vi "LoadPosMove.vi"(11 "UiDefinition":T1) -> ()   [LabVIEW 2020]
uses:
  UIReferences.ctl
  C:/Users/User/Desktop/Automation/CurrentVersion/LabviewDXFViewer/bin/Release/LabviewDXFViewer.exe
  LabviewDXFViewer/bin/Release/LabviewDXFViewer.exe
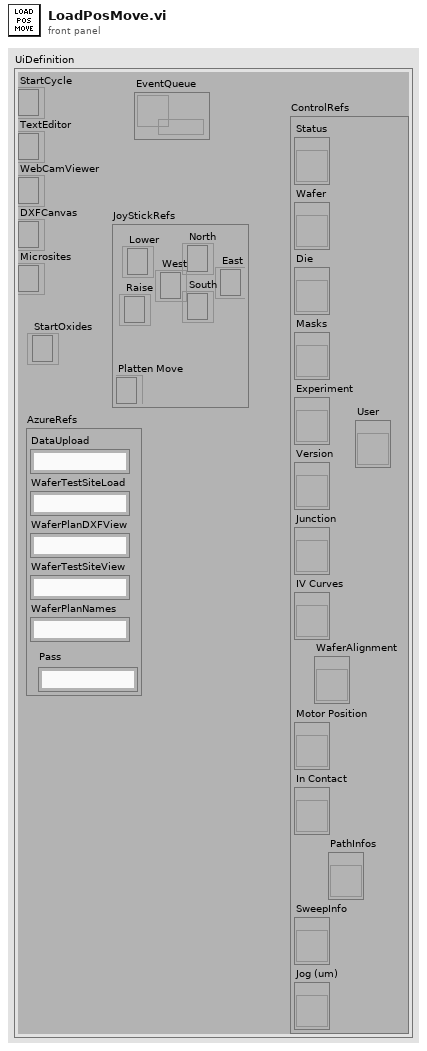
[diagram p1: front panel]
types:
  T1 = typedef "UIReferences.ctl" = cluster{"StartCycle":refnum<k24>, "TextEditor":refnum<k24>, "WebCamViewer":refnum<k24>, "DXFCanvas":refnum<k24>, "Microsites":refnum<k24>, "JoyStickRefs":cluster{"North":refnum<k24>, "Lower":refnum<k24>, "Raise":refnum<k24>, "Platten Move":refnum<k24>, "West":refnum<k24>, "East":refnum<k24>, "South":refnum<k24>}, "AzureRefs":cluster{"DataUpload":string, "WaferTestSiteLoad":string, "WaferPlanDXFView":string, "WaferTestSiteView":string, "WaferPlanNames":string, "Pass":string}, "ControlRefs":cluster{"Status":refnum<vi>, "Wafer":refnum<vi>, "Die":refnum<vi>, "Masks":refnum<vi>, "Experiment":refnum<vi>, "Version":refnum<vi>, "Junction":refnum<vi>, "IV Curves":refnum<vi>, "Motor Position":refnum<vi>, "In Contact":refnum<vi>, "SweepInfo":refnum<vi>, "Jog (um)":refnum<vi>, "PathInfos":refnum<vi>, "User":refnum<vi>, "WaferAlignment":refnum<vi>}, "EventQueue":refnum<queue>, "StartOxides":refnum<k24>}
  T2 = typedef "WaferAlignmentType.ctl" = cluster{"Wafer Units to microns":dbl, "Rotation Misalign":dbl[], "Scale Misalign":dbl, "Steps Per micron":dbl, "Position 1":i32[], "Position 2":i32[], "Lift Distance":i32, "Position 3":i32[], "Jog Height":i32}
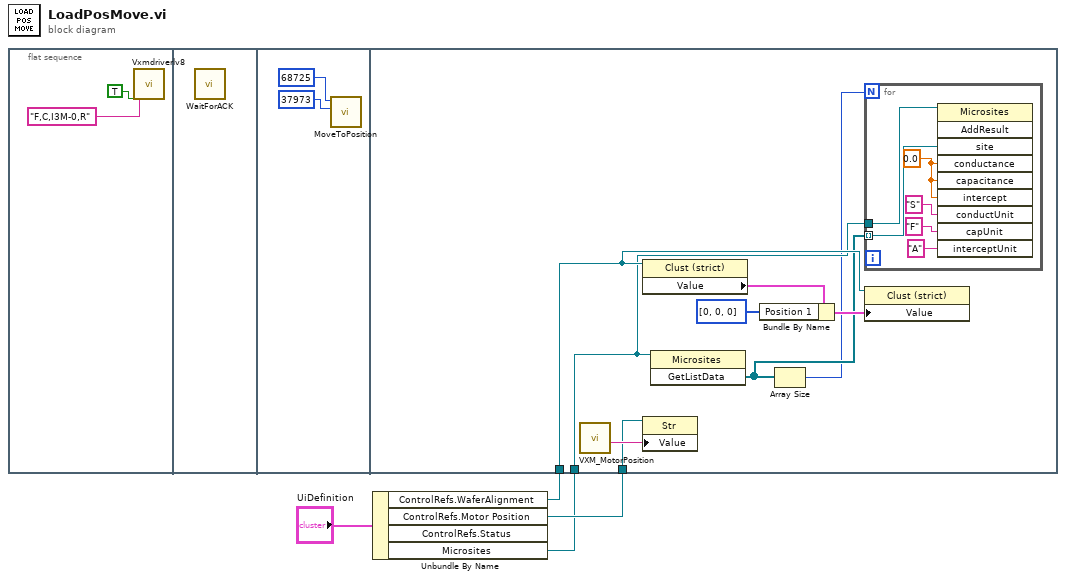
[diagram p0: block diagram]
diagram:
  n1 = flat-sequence {
    tunnel: w3 -> [w16]
    tunnel: w2 -> [w13]
    tunnel: w1 -> [w11]
    frame #0 {
      n2 = call "Vxmdriverlv8.Vi"("Send\nchars\nto port"=TRUE, "Chars to send"="F,C,I3M-0,R") -> ()  [unwired: 20 in, 6 out]
    }
    frame #1 {
      n3 = call "WaitForACK.vi"() -> ()  [unwired: 12 in]
    }
    frame #2 {
      n4 = call "MoveToPosition.vi"("Y"=37973 ("X"), "X"=68725 ("Y")) -> ()  [unwired: 10 in]
    }
    frame #3 {
      n5 = call "VXM_MotorPosition.vi"() -> ("Position String"=w17:string)  [unwired: 10 in, 1 out]
      n6 = property class="Clust (strict)"(reference=w13) -> ("Value"=w15:T2)  [unwired: 1 in, 2 out]
      n7 = property class="Str"(reference=w16, "Value"=w17) -> ()  [unwired: 1 in, 2 out]
      n8 = invoke class="Microsites" method="GetListData"(reference=w11) -> ("GetListData"=w10:refnum<k24>[])  [unwired: 2 in, 2 out]
      n9 = Bundle By Name(cluster=w15, "Position 1"=i32[] [0, 0, 0]) -> (w12:T2)
      n10 = Array Size(array=w10) -> (size(s)=w9:i32)
      n11 = for {
        N: w9 -> [_]
        tunnel: w11 -> [w20]
        tunnel: w10 -> [w18] mode=indexing
        w19 = 0.0 ("conductance")
        n12 = invoke class="Microsites" method="AddResult"(reference=w20, "site"=w18, "conductance"=w19, "capacitance"=w19, "intercept"=w19, "conductUnit"="S", "capUnit"="F", "interceptUnit"="A") -> ()  [unwired: 2 in, 10 out]
      }
      n13 = property class="Clust (strict)"(reference=w13, "Value"=w12) -> ()  [unwired: 1 in, 2 out]
    }
  }
  n14 = Unbundle By Name("UiDefinition") -> ("ControlRefs.WaferAlignment"=w2:refnum<vi>, "ControlRefs.Motor Position"=w3:refnum<vi>, "Microsites"=w1:refnum<k24>)  [unwired: 1 out]
